vi "Pump Water.vi"(8 "error in (no error)":errorcluster, 10 "enable?":bool, 11 "Swamp Cooler in":refnum<class "Evaporative Cooler.lvclass">) -> (0 "error out":errorcluster, 3 "Swamp Cooler out":refnum<class "Evaporative Cooler.lvclass">)   [LabVIEW 2023, in "Evaporative Cooler.lvclass"]
uses:
  Evaporative Cooler.lvclass
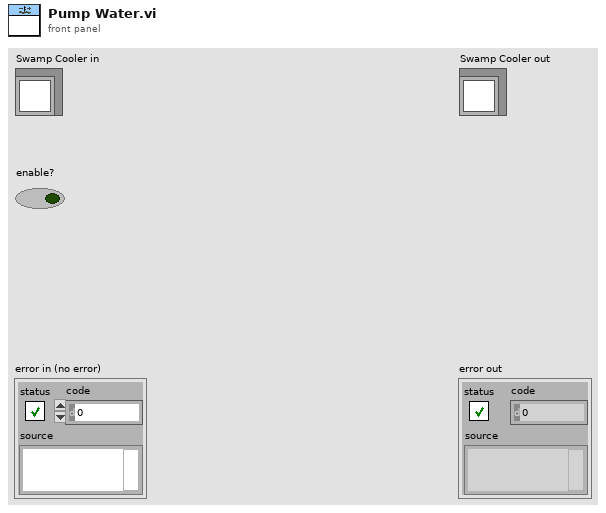
[diagram p1: front panel]
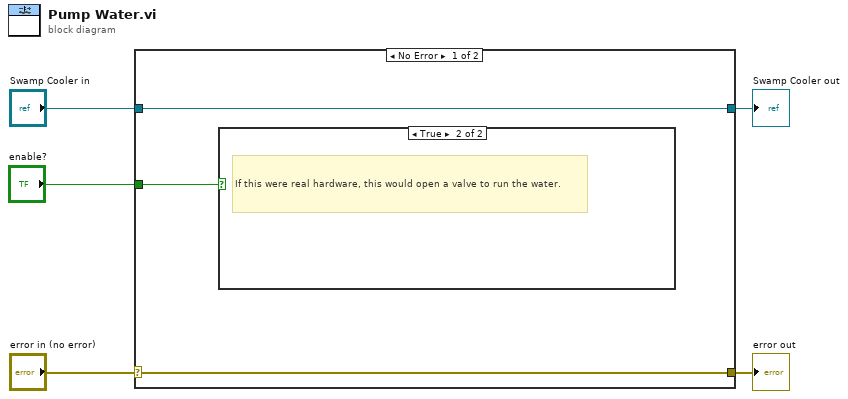
[diagram p0: block diagram]
diagram:
  n1 = case shown="No Error" "error in (no error)" {
    selector: "error in (no error)" -> [w7 w10]
    tunnel: [w7 w10] -> w4
    tunnel: [w8 w9] -> w2
    tunnel: "Swamp Cooler in" -> [w8 w9]
    tunnel: "enable?" -> [w6 _]
    frame No Error {
      n2 = case shown="True" w6 {
        frame False {
          # "If this were real hardware, this would close a valve to stop the water."
        }
        frame True {
          # "If this were real hardware, this would open a valve to run the water."
        }
      }
    }
    frame Error {
    }
  }
  "error out" <- w4
  "Swamp Cooler out" <- w2
